vi "FTW-SyncServer-Await.vi"(0 "FTW Synchronous Server":refnum<data-value>, 5 "Receive Timeout":i32=100 format="%dmsec", 11 "error in":errorcluster) -> (4 "FTW Synchronous Server out":refnum<data-value>, 6 "Incoming Request":string, 15 "error out":errorcluster)   [LabVIEW 2014]
uses:
  core/FTW-SyncServer-Core-Type.ctl
  error/FTW-ERR-ThrowGenericError.vi
  error/FTW-ERR-ThrowError.vi
  error/FTW-ERR-NoErrorConstant.vi
  error/FTW-ERR-CallChain.vi
  string/FTW-STR-ReplaceWhitespace.vi
panel:
  # "Inputs"
  # "Outputs"
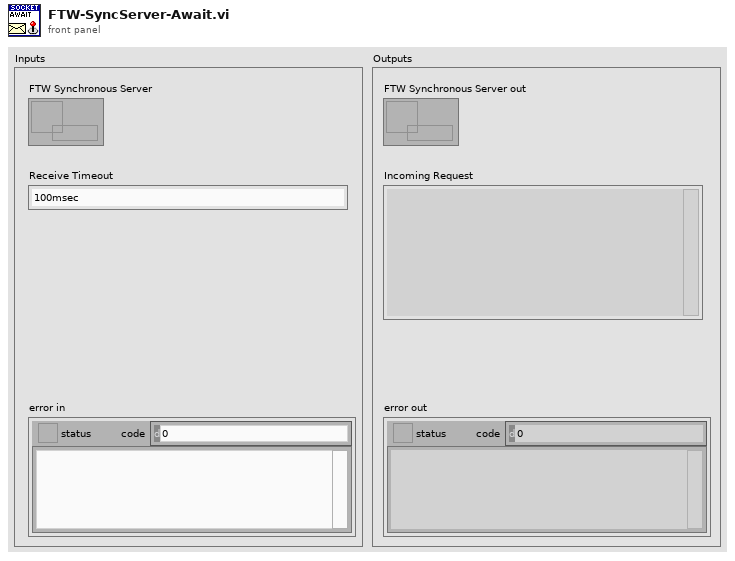
[diagram p1: front panel]
types:
  T1 = typedef "FTW-SyncServer-Core-Type.ctl" = cluster{"Socket":i64}
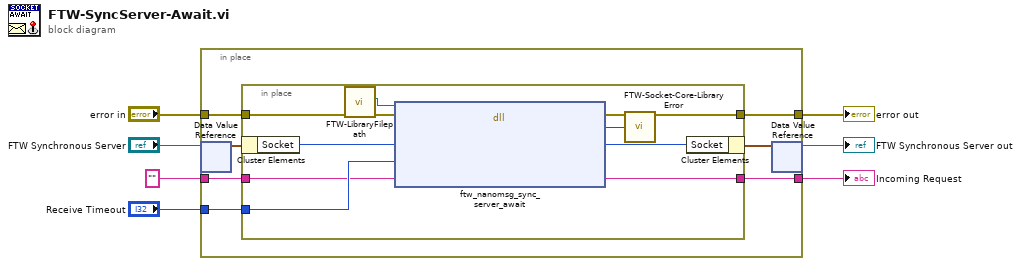
[diagram p0: block diagram]
diagram:
  n1 = in-place {
    in-place-border: "error in" -> [w14]
    in-place-border: [w13] -> w3
    in-place-border: "Receive Timeout" -> [w12]
    in-place-border: [w9] -> w4
    in-place-border: "" -> [w8]
    n2 = in-place-dvr #1("FTW Synchronous Server") -> (w11:T1)  [unwired: 1 out]
    n3 = in-place {
      in-place-border: w14 -> [w25]
      in-place-border: [w23] -> w13
      in-place-border: w12 -> [w20]
      in-place-border: [w16] -> w9
      in-place-border: w8 -> [w15]
      n4 = in-place-cluster #2(w11) -> ("Socket"=w18:i64)
      n5 = call "FTW-LibraryFilepath.vi"("error in"=w25) -> ("error out"=w21:errorcluster, "Library Filepath"=w22:path)  [unwired: 8 in, 1 out]
      n6 = dll-call lib="?" fn="ftw_nanomsg_sync_server_await"(path in=w22, error in=w21, "Socket Handle"=w18, "Recv Timeout"=w20, "Incoming Request"=w15) -> (error out=w24:errorcluster, "Return Value"=w19:i64, "Socket Handle"=w17:i64, "Incoming Request"=w16:string)  [unwired: 2 in, 1 out]
      n7 = call "FTW-Socket-Core-LibraryError.vi"("error in"=w24, "Return Value"=w19) -> ("error out"=w23:errorcluster)  [unwired: 13 in]
      n8 = in-place-cluster #2("Socket"=w17) -> (w10:T1)
    }
    n9 = in-place-dvr #1(w10) -> (→"FTW Synchronous Server out":refnum<data-value>)  [unwired: 1 out]
  }
  "error out" <- w3
  "Incoming Request" <- w4
